vi "Alarma_Tolerancia.vi"(6 "Tipo Señal":enum16{"Voltaje", "Frecuencia", "Voltaje AVG"}(ring), 7 "ID_EQUIPO":i32=1, 9 "Motivo Alarma":string="Tolerancia de Frecuencia en Generador 1", 10 "Señal in":sgl, 11 "timref in":refnum<data-value>) -> (2 "alarm":bool)   [LabVIEW 2018]
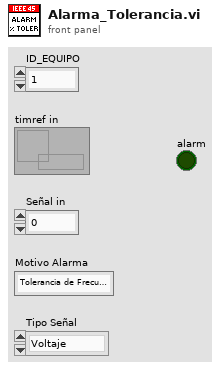
[diagram p1: front panel]
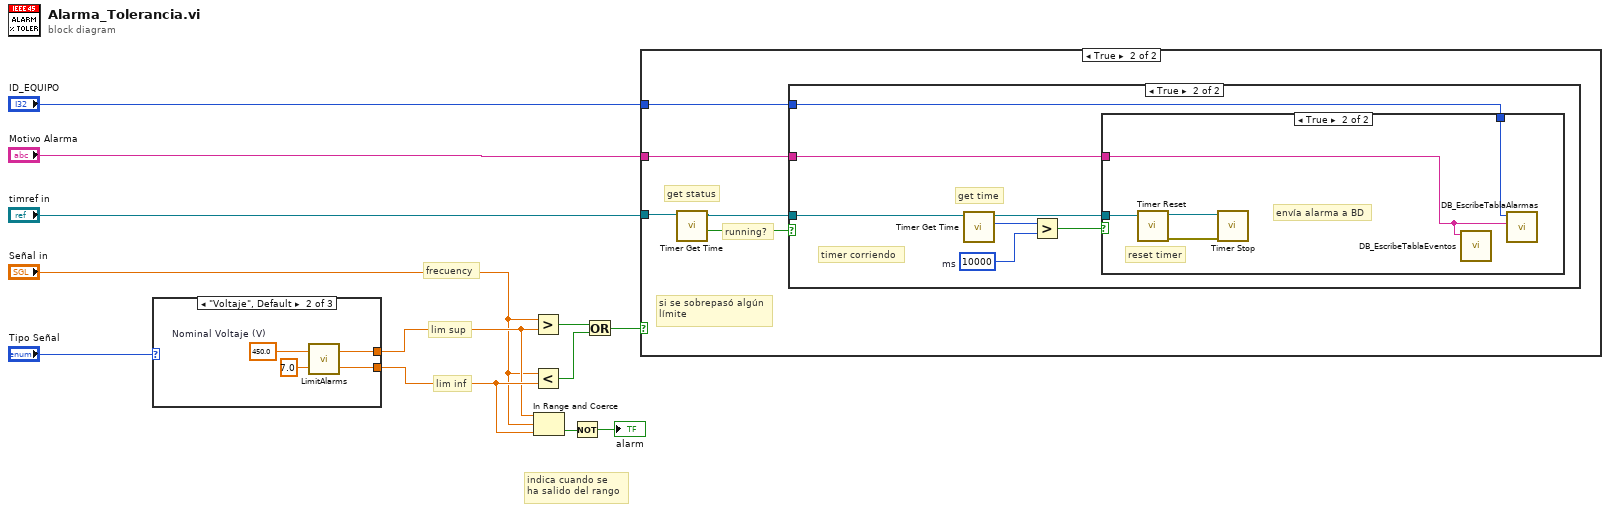
[diagram p0: block diagram]
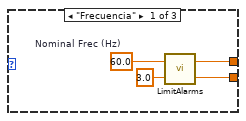
[diagram p2: hidden frame]
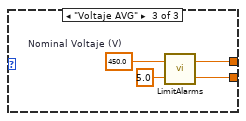
[diagram p3: hidden frame]
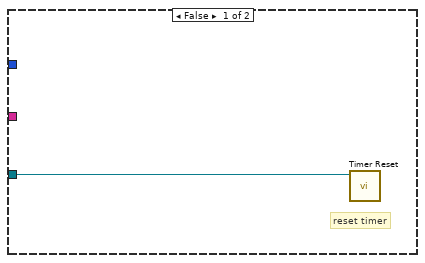
[diagram p4: hidden frame]
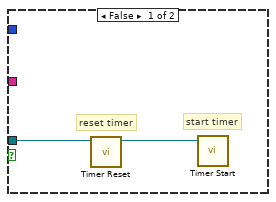
[diagram p5: hidden frame]
diagram:
  # "indica cuando se \nha salido del rango"
  # "lim inf"
  # "lim sup"
  # "frecuency"
  n1 = case shown="\"Voltaje\", Default" "Tipo Señal" {
    tunnel: [w16 w20 w24] -> w5
    tunnel: [w15 w19 w23] -> w4
    frame "Frecuencia" {
      w13 = sgl 60.0  # Nominal Frec (Hz)
      n2 = call "LimitAlarms.vi"("Value"=sgl 3.0, "Parameter"=w13) -> ("Min"=w16:sgl, "Max"=w15:sgl)
    }
    frame "Voltaje", Default {
      w17 = sgl 450.0  # Nominal Voltaje (V)
      n3 = call "LimitAlarms.vi"("Value"=sgl 7.0, "Parameter"=w17) -> ("Min"=w20:sgl, "Max"=w19:sgl)
    }
    frame "Voltaje AVG" {
      w21 = sgl 450.0  # Nominal Voltaje (V)
      n4 = call "LimitAlarms.vi"("Value"=sgl 5.0, "Parameter"=w21) -> ("Min"=w24:sgl, "Max"=w23:sgl)
    }
  }
  n5 = Greater?(x="Señal in", y=w4) -> (0:w11:bool)
  n6 = Less?(x="Señal in", y=w5) -> (x < y?=w10:bool)
  n7 = In Range and Coerce(upper limit=w4, x="Señal in", lower limit=w5) -> (In Range?=w2:bool)  [unwired: 1 out]
  n8 = Not(x=w2) -> (.not. x?=→"alarm":bool)
  n9 = Or(x=w11, y=w10) -> (x .or. y?=w12:bool)
  n10 = case shown="True" w12 {
    tunnel: "timref in" -> [w25 w30]
    tunnel: "Motivo Alarma" -> [_ w27]
    tunnel: "ID_EQUIPO" -> [_ w26]
    frame False {
      # "reset timer"
      n11 = call "Timer Reset.vi"("Timer reference"=w25) -> ()  [unwired: 9 in, 2 out]
    }
    frame True {
      # "get status"
      # "si se sobrepasó algún\nlímite"
      # "running?"
      n12 = call "Timer Get Time.vi"("Timer reference"=w30) -> ("Running ?"=w29:bool, "Timer reference  out"=w28:refnum<data-value>)  [unwired: 7 in, 2 out]
      n13 = case shown="True" w29 {
        tunnel: w28 -> [w32 w37]
        tunnel: w27 -> [_ w34]
        tunnel: w26 -> [_ w33]
        frame False {
          # "reset timer"
          # "start timer"
          n14 = call "Timer Reset.vi"("Timer reference"=w32) -> ("Timer reference  out"=w31:refnum<data-value>)  [unwired: 9 in, 1 out]
          n15 = call "Timer Start.vi"("Timer reference"=w31) -> ()  [unwired: 9 in, 2 out]
        }
        frame True {
          w38 = u32 10000  # ms
          # "timer corriendo"
          # "get time"
          n16 = call "Timer Get Time.vi"("Timer reference"=w37) -> ("Elapsed Time (ms)"=w39:u32, "Timer reference  out"=w35:refnum<data-value>)  [unwired: 7 in, 2 out]
          n17 = Greater?(x=w39, y=w38) -> (0:w36:bool)
          n18 = case shown="True" w36 {
            tunnel: w35 -> [_ w44]
            tunnel: w34 -> [_ w40]
            tunnel: w33 -> [_ w41]
            frame False {
              # "espera que se cumpla el tiempo"
            }
            frame True {
              # "envía alarma a BD"
              # "reset timer"
              n19 = call "Timer Reset.vi"("Timer reference"=w44) -> ("error out"=w42:errorcluster, "Timer reference  out"=w43:refnum<data-value>)  [unwired: 9 in]
              n20 = call "Timer Stop.vi"("error in (no error)"=w42, "Timer reference"=w43) -> ()  [unwired: 8 in, 2 out]
              n21 = call "DB_EscribeTablaEventos.vi"("DESCRIPCION"=w40) -> ()  [unwired: 10 in, 1 out]
              n22 = call "DB_EscribeTablaAlarmas.vi"("MOTIVO"=w40, "ID_EQUIPO"=w41) -> ()  [unwired: 9 in, 1 out]
            }
          }
        }
      }
    }
  }
